vi "DataRefGet-禁用.vi"(8 "error in (no error)":errorcluster caption="错误输入（无错误）", 11 "MainPage 输入":refnum<class "MainPage.lvclass">) -> (0 "error out":errorcluster caption="错误输出", 1 "非法引用句柄？":bool, 2 "通讯接口记录":T1, 3 "MainPage 输出":refnum<class "MainPage.lvclass">, 4 "数据记录引用":refnum<data-value>)   [LabVIEW 2019, in "MainPage.lvlib" / "MainPage.lvclass"]
uses:
  MainPage.lvclass
panel:
  # "弃用，会闪退"
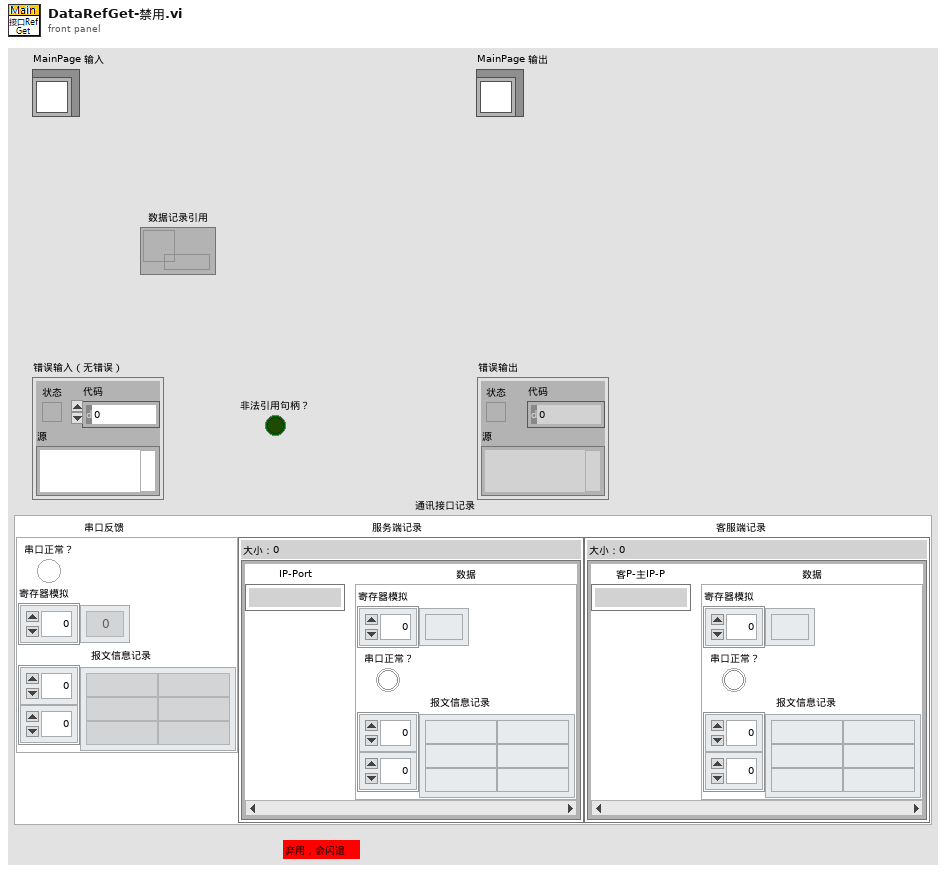
[diagram p1: front panel]
types:
  T1 = typedef "MainPage.lvlib/MainPage.lvclass/DataRef_通讯接口数据记录-弃用.ctl" = cluster{"串口反馈":cluster{"串口正常？":bool, "寄存器模拟":u16[], "报文信息记录":string[][]}, "服务端记录":map{string, cluster{"寄存器模拟":u16[], "串口正常？":bool, "报文信息记录":string[][]}}, "客服端记录":map{string, cluster{"寄存器模拟":u16[], "串口正常？":bool, "报文信息记录":string[][]}}}
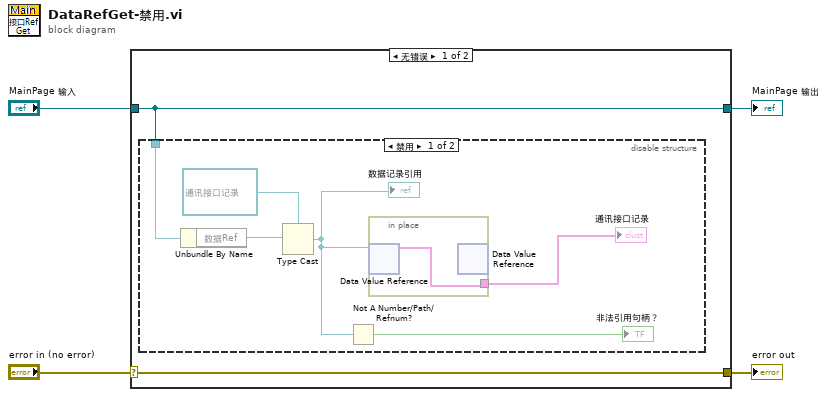
[diagram p0: block diagram]
diagram:
  n1 = case shown="无错误" "error in (no error)" {
    selector: "error in (no error)" -> [w6 w15]
    tunnel: [w6 w15] -> w3
    tunnel: [w5 w14] -> w1
    tunnel: "MainPage 输入" -> [w5 w14]
    frame No Error {
      n2 = disable-structure shown="禁用" {
        disable-tunnel: w5 -> [w12 _]
        frame Disabled {
          n3 = Unbundle By Name(w12) -> ("数据Ref"=w9:u32)
          n4 = Type Cast(type=refnum<data-value> refnum ("数据记录引用"), x=w9) -> (*(type *) &x=w10:refnum<data-value>)
          "数据记录引用" <- w10
          n5 = Not A Number/Path/Refnum?(number/path/refnum=w10) -> (NaN/Path/Refnum?=→"非法引用句柄？":bool)
          n6 = in-place {
            in-place-border: [w13] -> w7
            n7 = in-place-dvr #1(w10) -> (w13:T1)  [unwired: 1 out]
            n8 = in-place-dvr #1() -> ()  [unwired: 1 in, 2 out]
          }
          "通讯接口记录" <- w7
        }
        frame Enabled {
        }
      }
    }
    frame Error {
    }
  }
  "error out" <- w3
  "MainPage 输出" <- w1
